vi "clean.vi"(8 "error in (no error)":errorcluster) -> (0 "error out":errorcluster, 3 "CNT90 out":refnum<class "CNT90.lvclass">)   [LabVIEW 2019, in "CNT90.lvclass"]
uses:
  CNT90.lvclass
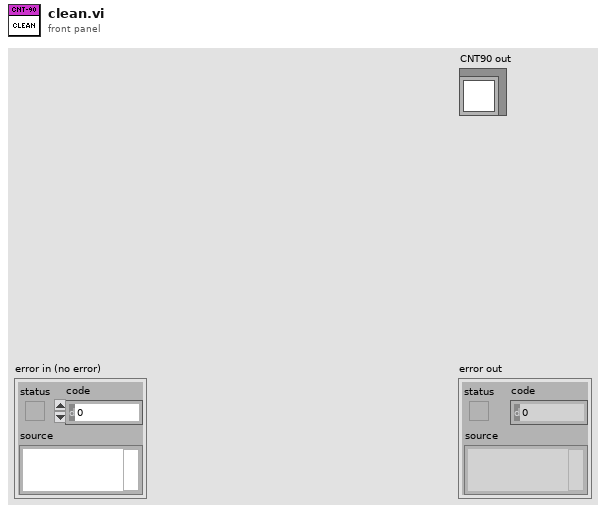
[diagram p1: front panel]
types:
  T1 = cluster{"error":bool, "code":i32, "source":string}
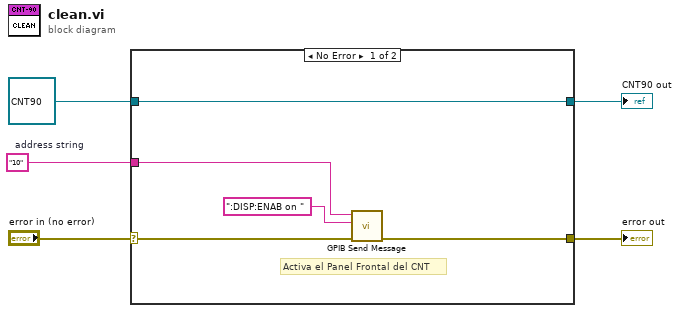
[diagram p0: block diagram]
diagram:
  w1 = "10"  # address string
  n1 = case shown="No Error" "error in (no error)" {
    selector: "error in (no error)" -> [w8 w12]
    tunnel: [w7 w12] -> w4
    tunnel: [w10 w11] -> w2
    tunnel: refnum<class "CNT90.lvclass"> refnum ("CNT90 in") -> [w10 w11]
    tunnel: w1 -> [w6 _]
    frame No Error {
      # "Activa el Panel Frontal del CNT"
      n2 = call <instrlib>:"GPIB Send Message.vi"("address string"=w6, "write buffer"=":DISP:ENAB on ", "error in"=w8) -> ("error out"=w7:T1)  [unwired: 4 in, 2 out]
    }
    frame Error {
    }
  }
  "error out" <- w4
  "CNT90 out" <- w2
